vi "get Tx Rx Result.vi"(10 "result":i32, 11 "protocol_version":i32) -> (3 "function return":string)   [LabVIEW 2016, in "dxl_x86_c.lvlib"]
doc: "WINDECLSPEC const char *getTxRxResult (int protocol_version, int result);"
uses:
  dxl_x86_c.lvlib
  dxl_x86_c.dll
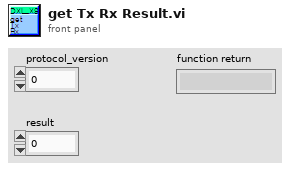
[diagram p1: front panel]
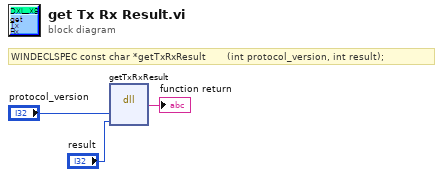
[diagram p0: block diagram]
diagram:
  # "WINDECLSPEC const char *getTxRxResult       (int protocol_version, int result);"
  n1 = dll-call lib="C:/Users/Platform/Desktop/DynamixelSDK/labview/dxl_x86_c.lvlib/dxl_x86_c.*" fn="getTxRxResult"("protocol_version"="protocol_version", "result"="result") -> (→"function return":string)  [unwired: 5 in, 2 out]
